vi "Thermometer (Demo).vi"(10 "Units (0: Celsius)":u16(ring) items=["Celsius", "Fahrenheit"]) -> (1 "Temperature Value":dbl(slide) scale=0.0..100.0)   [LabVIEW 2017]
doc: "This VI simulates measuring a temperature using the temperature sensor on the DAQ BNC-2120 terminal block.\n\nIf you have a DAQ board connected to the BNC-2120 and have configured the system in MAX, then use the Thermometer VI instead."
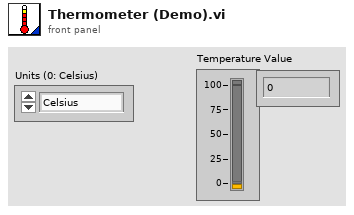
[diagram p1: front panel]
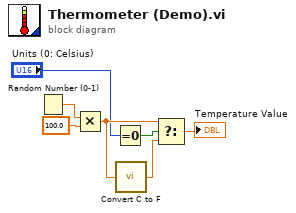
[diagram p0: block diagram]
diagram:
  n1 = Random Number (0-1)() -> (number: 0 to 1=w1:dbl)
  n2 = Multiply(x=w1, y=100.0) -> (x*y=w5:dbl)
  n3 = Equal To 0?(x="Units (0: Celsius)") -> (x = 0?=w2:bool)
  n4 = call "Convert C to F.vi"("Degrees Celsius"=w5) -> ("Degrees Fahrenheit"=w7:dbl)
  n5 = Select(t=w5, s=w2, f=w7) -> (s? t:f=→"Temperature Value":dbl)
